vi "VariableWriteArray.vi"() -> ()   [LabVIEW 2009]
panel:
  out "Writing":bool
  in  "stop":bool
  out "Data Array":dbl[](array[numeric])
  out "Numeric":i32
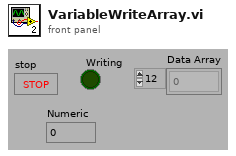
[diagram p1: front panel]
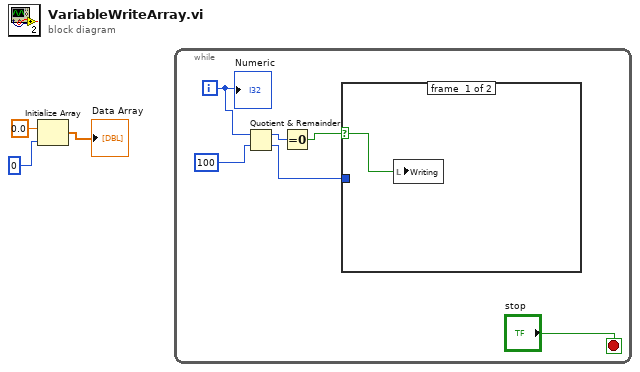
[diagram p0: block diagram]
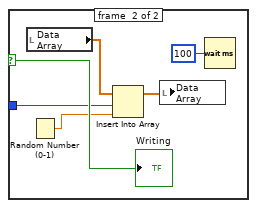
[diagram p2: hidden frame]
diagram:
  n1 = Initialize Array(0.0 ("element"), 0 ("dimension size")) -> (→"Data Array":dbl[])
  n2 = while {
    i -> [w7]
    stop <- "stop" stop-if-true
    n3 = Quotient & Remainder(x=w7, y=100) -> (x-y*floor(x/y)=w6:i32, floor(x/y)=w4:i32)
    n4 = Equal To 0?(x=w6) -> (x = 0?=w5:bool)
    n5 = case shown="True" w5 {
      selector: w5 -> [w10 w16]
      tunnel: w4 -> [_ w14]
      frame #0 {
        n6 = local write "Writing"(w10) -> ()
      }
      frame #1 {
        n7 = local read "Data Array"() -> (w11:dbl[])
        n8 = Random Number (0-1)() -> (number: 0 to 1=w15:dbl)
        n9 = Insert Into Array(array=w11, index=w14, new element=w15) -> (w12:dbl[])
        n10 = local write "Data Array"(w12) -> ()
        n11 = Wait (ms)(milliseconds to wait=u32 100) -> ()  [unwired: 1 out]
        "Writing" <- w16
      }
    }
    "Numeric" <- w7
  }
